vi "TWM Parse Session Parameters for Phase.vi"(8 "error in":errorcluster, 10 "phase index (1: default)":i32=1, 11 "TWM session items":T2) -> (0 "error out":errorcluster, 3 "TWM channel info":T1)   [LabVIEW 2013]
doc: "Extract given phase data from loaded TWM session."
uses:
  TWM Session Data.ctl
  TWM Phase Info.ctl
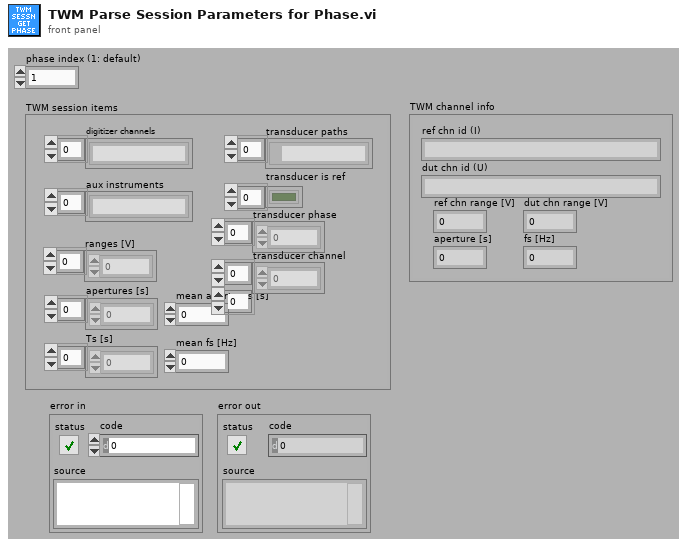
[diagram p1: front panel]
types:
  T1 = typedef "TWM Phase Info.ctl" = cluster{"ref chn id (I)":string, "dut chn id (U)":string, "ref chn range [V]":dbl, "dut chn range [V]":dbl, "aperture [s]":dbl, "fs [Hz]":dbl}
  T2 = typedef "TWM Session Data.ctl" = cluster{"digitizer channels":string[], "aux instruments":string[], "ranges [V]":dbl[], "apertures [s]":dbl[], "Ts [s]":dbl[], "mean apertures [s]":dbl, "mean fs [Hz]":dbl, "transducer paths":path[], "transducer is ref":bool[], "transducer phase":i32[], "transducer channel":i32[][]}
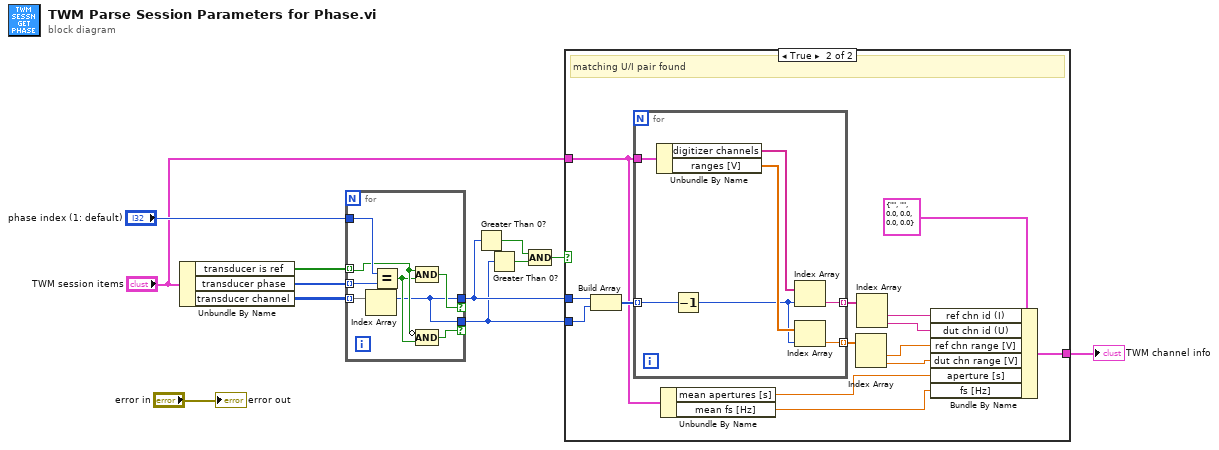
[diagram p0: block diagram]
diagram:
  n1 = Unbundle By Name("TWM session items") -> ("transducer is ref"=w12:bool[], "transducer phase"=w11:i32[], "transducer channel"=w1:i32[][])
  n2 = for {
    tunnel: w12 -> [w17] mode=indexing
    tunnel: w11 -> [w20] mode=indexing
    tunnel: w1 -> [w15] mode=indexing
    tunnel: "phase index (1: default)" -> [w19]
    tunnel: [w13] -> w5 if=w18
    tunnel: [w13] -> w4 if=w14
    n3 = Index Array(array=w15) -> (element=w13:i32)  [unwired: 1 in]
    n4 = Equal?(x=w19, y=w20) -> (x = y?=w16:bool)
    n5 = Compound Arithmetic op=AND(w17, w16) -> (w18:bool)
    n6 = Compound Arithmetic op=AND(invert w17, w16) -> (w14:bool)
  }
  n7 = Greater Than 0?(x=w5) -> (x > 0?=w7:bool)
  n8 = Greater Than 0?(x=w4) -> (x > 0?=w8:bool)
  n9 = Compound Arithmetic op=AND(w7, w8) -> (w6:bool)
  n10 = case shown="True" w6 {
    tunnel: w5 -> [_ w34]
    tunnel: w4 -> [_ w33]
    tunnel: "TWM session items" -> [_ w24]
    tunnel: [_ w21] -> w2
    frame False {
    }
    frame True {
      # "matching U/I pair found"
      n11 = Build Array(w34, w33) -> (w32:i32[])
      n12 = for {
        tunnel: w32 -> [w38] mode=indexing
        tunnel: w24 -> [w41]
        tunnel: [w37] -> w31 mode=indexing
        tunnel: [w36] -> w30 mode=indexing
        n13 = Unbundle By Name(w41) -> ("digitizer channels"=w40:string[], "ranges [V]"=w39:dbl[])
        n14 = Decrement(x=w38) -> (x-1=w35:i32)
        n15 = Index Array(array=w40, index=w35) -> (element=w37:string)
        n16 = Index Array(array=w39, index=w35) -> (element=w36:dbl)
      }
      n17 = Unbundle By Name(w24) -> ("mean apertures [s]"=w23:dbl, "mean fs [Hz]"=w22:dbl)
      n18 = Index Array(array=w30) -> (element #1=w26:dbl, element #2=w25:dbl)  [unwired: 2 in]
      n19 = Index Array(array=w31) -> (element #1=w28:string, element #2=w27:string)  [unwired: 2 in]
      n20 = Bundle By Name(cluster=T1 {"ref chn id (I)"="", "dut chn id (U)"="", "ref chn range [V]"=0.0, "dut chn range [V]"=0.0, "aperture [s]"=0.0, "fs [Hz]"=0.0} ("TWM channel info"), "ref chn id (I)"=w28, "dut chn id (U)"=w27, "ref chn range [V]"=w26, "dut chn range [V]"=w25, "aperture [s]"=w23, "fs [Hz]"=w22) -> (w21:T1)
    }
  }
  "TWM channel info" <- w2
  "error out" <- "error in"
